vi "0MQ_Server.TestReply.vi"() -> ()   [LabVIEW 2014, in "0MQ_Server.lvclass"]
uses:
  0MQ_Server.lvclass
  <vilib>/JKI/JKI SMO/SMO/Typedefs/SMOState --Enum.ctl
  Typedefs/Socket Config.ctl
  <vilib>/addons/zeromq/socket_type.ctl
  0MQ_Server.lvclass/0MQ_Server.ctl
  <vilib>/JKI/JKI SMO/SMO/SMO.lvclass
  <vilib>/addons/zeromq/zeromq.lvlib
panel:
  in  "Reply Message":string="Reply"
  in  "Socket Filter":string
  out "incoming message":cluster{"identity":string, "data":string[]}
  out "SMO State":T1
  out "error out":errorcluster
  in  "Stop":bool
  # "SMO ZMQ REPLY"
  # "For instructions on how to use the JKI State Machine Objects, examples and video tutorials, visit:\nhttp://jki.net/state-machine-objects/\n\nJKI State Machine Objects™\nhttp://jki.net/state-machine-objects/\nCopyright (C) 2005-2015, JKI <info@jki.net>\nALL RIGHTS RESERVED"
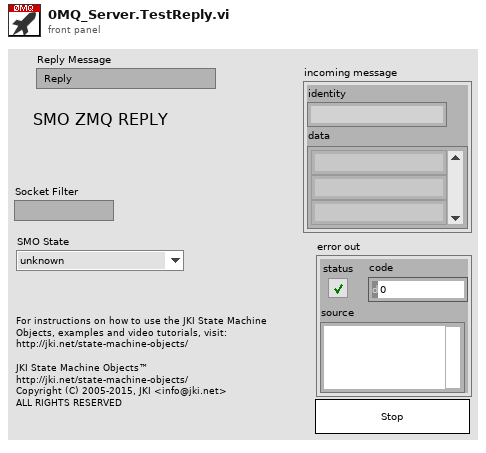
[diagram p1: front panel]
types:
  T1 = typedef "SMO.lvclass/SMOState --Enum.ctl" = enum16{"unknown", "Created", "Started", "Stopped"}
  T2 = typedef "0MQ_Server.lvclass/Socket Config.ctl" = cluster{"Socket type":T3, "endpoint":string, "socket filter":string}
  T3 = typedef "zeromq.lvlib/socket_type.ctl" = enum8{"ZMQ_PAIR", "ZMQ_PUB", "ZMQ_SUB", "ZMQ_REQ", "ZMQ_REP", "ZMQ_DEALER", "ZMQ_ROUTER", "ZMQ_PULL", "ZMQ_PUSH", "ZMQ_XPUB", "ZMQ_XSUB"}
  T4 = typedef "SMO.lvclass/Public Events.ctl" = cluster{"Error":refnum<user-event>, "State":refnum<user-event>}
  T5 = typedef "0MQ_Server.lvclass/0MQ_Server.PublicEvents.ctl" = cluster{"Incoming Message":refnum<user-event>}
  T6 = cluster{"Event Registration Refnum":refnum<event-registration>}
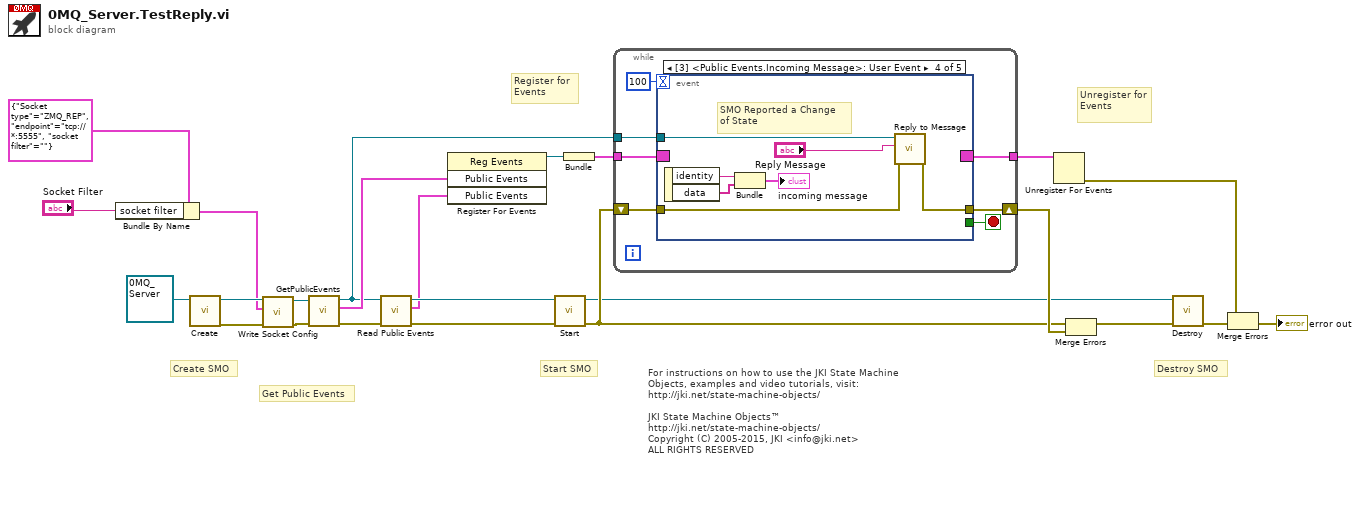
[diagram p0: block diagram]
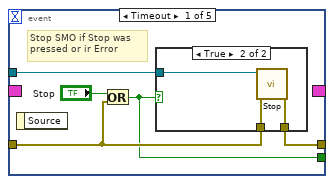
[diagram p2: hidden frame]
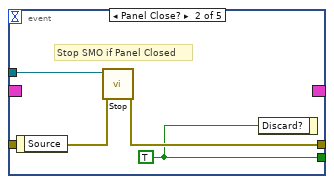
[diagram p4: hidden frame]
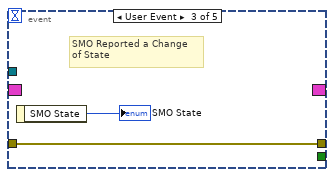
[diagram p5: hidden frame]
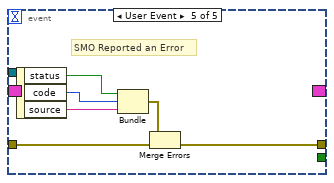
[diagram p6: hidden frame]
diagram:
  # "For instructions on how to use the JKI State Machine Objects, examples and video tutorials, visit:\nhttp://jki.net/state-machine-objects/\n\nJKI State Machine Objects™\nhttp://jki.net/state-machine-objects/\nCopyright (C) 2005-2015, JKI <info@jki.net>\nALL RIGHTS RESERVED"
  # "Get Public Events"
  # "Start SMO"
  # "Destroy SMO"
  # "Create SMO"
  # "Unregister for Events"
  # "Register for Events"
  n1 = Bundle By Name(cluster=T2 {"Socket type"=enum."ZMQ_REP", "endpoint"="tcp://*:5555", "socket filter"=""} ("Socket Config"), "socket filter"="Socket Filter") -> (w6:T2)
  n2 = call <vilib>:"Create.vi"("SMO"=refnum<class "0MQ_Server.lvclass"> refnum ("SMO.Template.lvclass")) -> ("error out"=w9:errorcluster, "SMO out"=w12:refnum<class "0MQ_Server.lvclass">)  [unwired: 9 in]
  n3 = call "Write Socket Config.vi"("error in (no error)"=w9, "Socket Config"=w6, "0MQ_Server in"=w12) -> ("error out"=w10:errorcluster, "0MQ_Server out"=w11:refnum<class "0MQ_Server.lvclass">)  [unwired: 7 in]
  n4 = call <vilib>:"GetPublicEvents.vi"("error in (no error)"=w10, "SMO"=w11) -> ("error out"=w3:errorcluster, "Public Events"=w14:T4, "SMO out"=w5:refnum<class "0MQ_Server.lvclass">)  [unwired: 7 in]
  n5 = call "Read Public Events.vi"("error in (no error)"=w3, "0MQ_Server in"=w5) -> ("error out"=w2:errorcluster, "Public Events"=w1:T5, "0MQ_Server out"=w4:refnum<class "0MQ_Server.lvclass">)  [unwired: 7 in]
  n6 = register-events(w14, w1) -> (reference out=w13:refnum<event-registration>)  [unwired: 2 in, 1 out]
  n7 = call <vilib>:"Start.vi"("error in (no error)"=w2, "SMO"=w4) -> ("error out"=w17:errorcluster, "SMO out"=w15:refnum<class "0MQ_Server.lvclass">)  [unwired: 8 in]
  n8 = Bundle("Event Registration Refnum"=w13) -> (w23:T6)  [unwired: 1 in]
  n9 = while {
    shift-right: [w30] -> w22
    shift-left: w17 -> [w29]
    tunnel: w23 -> [w28]
    tunnel: [w27] -> w24
    tunnel: w5 -> [w26]
    stop <- w31 stop-if-true
    n10 = event shown="[3] <Public Events.Incoming Message>: User Event" {
      selector: w28 -> [_ _ _ _ _]
      dyn-events: [_ _ _ _ _] -> w27
      timeout: 100 -> [_ _ _ _ _]
      tunnel: [w32 w41 _ _ _] -> w31
      tunnel: w26 -> [w36 w44 _ w50 _]
      tunnel: [w35 w43 w46 w48 w55] -> w30
      tunnel: w29 -> [w34 w42 w46 w49 w56]
      event Timeout {
        # "Stop SMO if Stop was \npressed or ir Error"
        n11 = event-data() -> ()  [unwired: 1 in, 1 out]
        n12 = Or(x="Stop", y=w34) -> (x .or. y?=w32:bool)
        n13 = case shown="True" w32 {
          tunnel: w36 -> [_ w40]
          tunnel: [w37 w39] -> w35
          tunnel: w34 -> [w37 w38]
          frame False {
          }
          frame True {
            n14 = call <vilib>:"Stop.vi"("error in (no error)"=w38, "SMO"=w40) -> ("error out"=w39:errorcluster)  [unwired: 8 in, 1 out]
          }
        }
      }
      event Panel Close? {
        w41 = TRUE ("OK")
        # "Stop SMO if Panel Closed"
        n15 = event-data() -> ()  [unwired: 1 in, 1 out]
        n16 = call <vilib>:"Stop.vi"("error in (no error)"=w42, "SMO"=w44) -> ("error out"=w43:errorcluster)  [unwired: 8 in, 1 out]
        n17 = event-data("Discard?"=w41) -> ()  [unwired: 1 in, 1 out]
      }
      event User Event {
        # "SMO Reported a Change\nof State"
        n18 = event-data() -> ("SMO State"=→"SMO State":T1)  [unwired: 1 in]
      }
      event User Event {
        # "SMO Reported a Change\nof State"
        n19 = event-data() -> ("identity"=w53:string, "data"=w52:string[])  [unwired: 1 in]
        n20 = Bundle("identity"=w53, "data"=w52) -> (→"incoming message":cluster{"identity":string, "data":string[]})  [unwired: 1 in]
        n21 = call-dynamic "Reply to Message.vi"("error in (no error)"=w49, "Message"="Reply Message", "0MQ_Server in"=w50) -> ("error out"=w48:errorcluster)  [unwired: 7 in, 1 out]
      }
      event User Event {
        # "SMO Reported an Error"
        n22 = event-data() -> ("status"=w54:bool, "code"=w58:i32, "source"=w57:string)  [unwired: 1 in]
        n23 = Bundle("status"=w54, "code"=w58, "source"=w57) -> (w59:errorcluster)  [unwired: 1 in]
        n24 = Merge Errors(w59, w56) -> (w55:errorcluster)
      }
    }
  }
  n25 = Unregister For Events(event registration refnum=w24) -> (error out=w21:errorcluster)  [unwired: 1 in]
  n26 = Merge Errors(w17, w22) -> (w16:errorcluster)
  n27 = call <vilib>:"Destroy.vi"("error in (no error)"=w16, "SMO"=w15) -> ("error out"=w19:errorcluster)  [unwired: 9 in]
  n28 = Merge Errors(w21, w19) -> (→"error out":errorcluster)
